vi "Projectile.vi"() -> ()   [LabVIEW 2014]
doc: "This program determines the range of a projectile launched at an angle. With a given launch speed and launch height, it displays a graph of range vs. angle (in degrees; from 0 to 90).\n\nBryan Ghahremani - SID: 1135515\nKenneth Heide - SID: 1269429"
uses:
  <vilib>/imath/engines/lvmath2/RunTimeEngine/Managers/WorkSpace/UID Generator.vi
  <vilib>/imath/engines/lvmath2/RunTimeEngine/RunTimeType/NIMS_RunTimeType_From StrictType (excl LVString).vi
  <instcachedir>/0/NIMS_RunTimeType_From StrictType (excl LVString)_15A5391EEA9C4AACB9955AC755B83D29.lvgen/NIMS_RunTimeType_From StrictType (excl LVString)_15A5391EEA9C4AACB9955AC755B83D29_000.vi
  <vilib>/imath/engines/lvmath2/RunTimeEngine/LocalVariableDefStatement/MC_LocalVariableDefStatement_Display.vi
  <vilib>/imath/engines/lvmath2/RunTimeEngine/BuiltInFunctions/power/NIMS_power.vi
  <instcachedir>/0/NIMS_power_EE9E8CEF339E4127BBD7FB98019394C4.lvgen/NIMS_power_EE9E8CEF339E4127BBD7FB98019394C4_017.vi
  <instcachedir>/0/NIMS_power_EE9E8CEF339E4127BBD7FB98019394C4.lvgen/NIMS_power_EE9E8CEF339E4127BBD7FB98019394C4_018.vi
  <vilib>/imath/engines/lvmath2/RunTimeEngine/ArithmeticOperatorToken/NIMS_ArithmeticOperator_plus.vi
  <instcachedir>/0/NIMS_ArithmeticOperator_plus_48D6EAACA5D645B09F7EC9C016C2DEA8.lvgen/NIMS_ArithmeticOperator_plus_48D6EAACA5D645B09F7EC9C016C2DEA8_001.vi
  <instcachedir>/0/NIMS_ArithmeticOperator_plus_48D6EAACA5D645B09F7EC9C016C2DEA8.lvgen/NIMS_ArithmeticOperator_plus_48D6EAACA5D645B09F7EC9C016C2DEA8_005.vi
  <vilib>/imath/engines/lvmath2/RunTimeEngine/ErrorHandling/NIMS_Create Error From Enums.vi
  <vilib>/imath/engines/lvmath2/RunTimeEngine/Managers/SymbolTable/Clear UID.vi
  <vilib>/imath/engines/lvmath2/RunTimeEngine/NodeEndStatement/NIMS_NodeEndStatement_Output.vi
  <instcachedir>/0/NIMS_NodeEndStatement_Output_53EC0D466D134D7ABD903AC30B43404B.lvgen/NIMS_NodeEndStatement_Output_53EC0D466D134D7ABD903AC30B43404B_005.vi
  <instcachedir>/0/NIMS_NodeEndStatement_Output_53EC0D466D134D7ABD903AC30B43404B.lvgen/NIMS_NodeEndStatement_Output_53EC0D466D134D7ABD903AC30B43404B_004.vi
  <vilib>/imath/engines/lvmath2/RunTimeEngine/ErrorHandling/NIMS_Finalize Error.vi
  <vilib>/imath/engines/lvmath2/RunTimeEngine/Managers/SymbolTable/NIMS_WorkSpace.lvlib
panel:
  out "XY Graph":cluster{"theta":i32[], "R":dbl[]}(graph)
  in  "Launch Height (m)":dbl
  in  "Launch Speed (m/s)":dbl
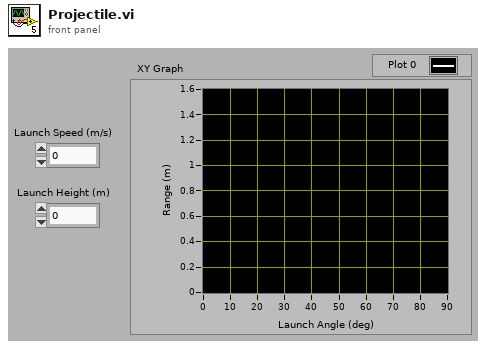
[diagram p1: front panel]
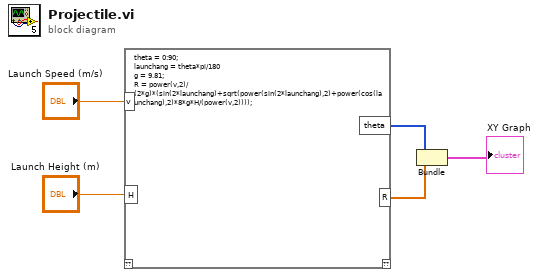
[diagram p0: block diagram]
diagram:
  n1 = mathscript code="theta = 0:90;\nlaunchang = theta*pi/180\ng = 9.81;\nR = power(v,2)/(2*g)*(sin(2*launchang)+sqrt(power(sin(2*launchang),2)+power(cos(launchang),2)*8*g*H/(power(v,2))));"("v"="Launch Speed (m/s)", "H"="Launch Height (m)") -> ("theta"=w5:i32[], "R"=w4:dbl[])  [unwired: 1 in, 1 out]
  n2 = Bundle("theta"=w5, "R"=w4) -> (→"XY Graph":cluster{"theta":i32[], "R":dbl[]})  [unwired: 1 in]
